vi "CAL_PRESSURE_TRANSDUCER 2016.vi"(7 "Array in":refnum<k24>[](array[refnum]), 8 "error in (no error)":errorcluster, 9 "Descriptions":string[](array[string]), 10 "Sensor Cluster":T1, 11 "pressure_slope_IN":dbl=51.35 format="%.2f") -> (0 "error out":errorcluster, 2 "Sensor Cluster 2":T1, 3 "pressure_slope_OUT":dbl=51.35 format="%.2f", 5 "Array out":refnum<k24>[](array[refnum]))   [LabVIEW 2016]
uses:
  controls/MCC DAQ Readings.ctl
  C:/Program Files (x86)/National Instruments/LabVIEW 2016/vi.lib/ULx/ULx_LV.dll
  Global_SIM_switch.vi
  Kpro Globals.vi
panel:
  out "ok":bool
  out "zero":bool
  out "Pressure":dbl format="%.2f"
  in  "ok":bool
  in  "zero":bool
  # "PRESSURE TRANSDUCER CALIBRATION"
  # "(step 1)"
  # "Fill graduated cylinder to 750 mL water.\nSubmerge Kpro effluent and start flow.\nStop flow at 800 mL of water (1 foot).\nAllow pressure to equilibrate and press zero."
  # "(step 2)"
  # "Hold Kpro effluent facing up and 5' above the floor.\nTurn Kpro flow on briefly to fill the Kpro line.\nTurn Kpro flow off again.\nPress OK when pressure has equilibrated"
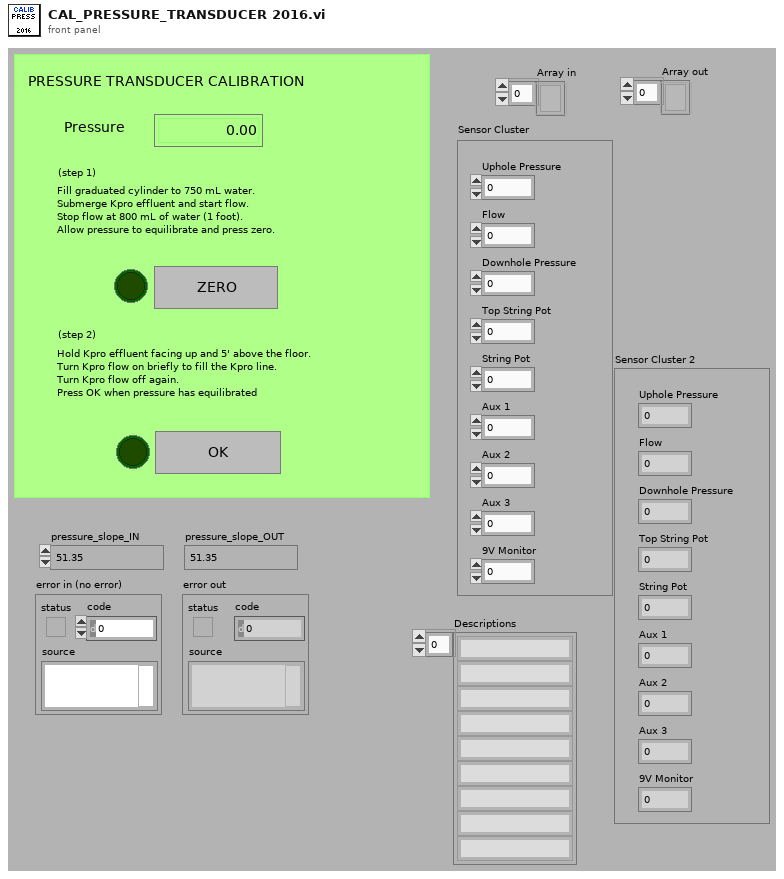
[diagram p1: front panel]
types:
  T1 = typedef "MCC DAQ Readings.ctl" = cluster{"Uphole Pressure":dbl, "Flow":dbl, "Downhole Pressure":dbl, "Top String Pot":dbl, "String Pot":dbl, "Aux 1":dbl, "Aux 2":dbl, "Aux 3":dbl, "9V Monitor":dbl}
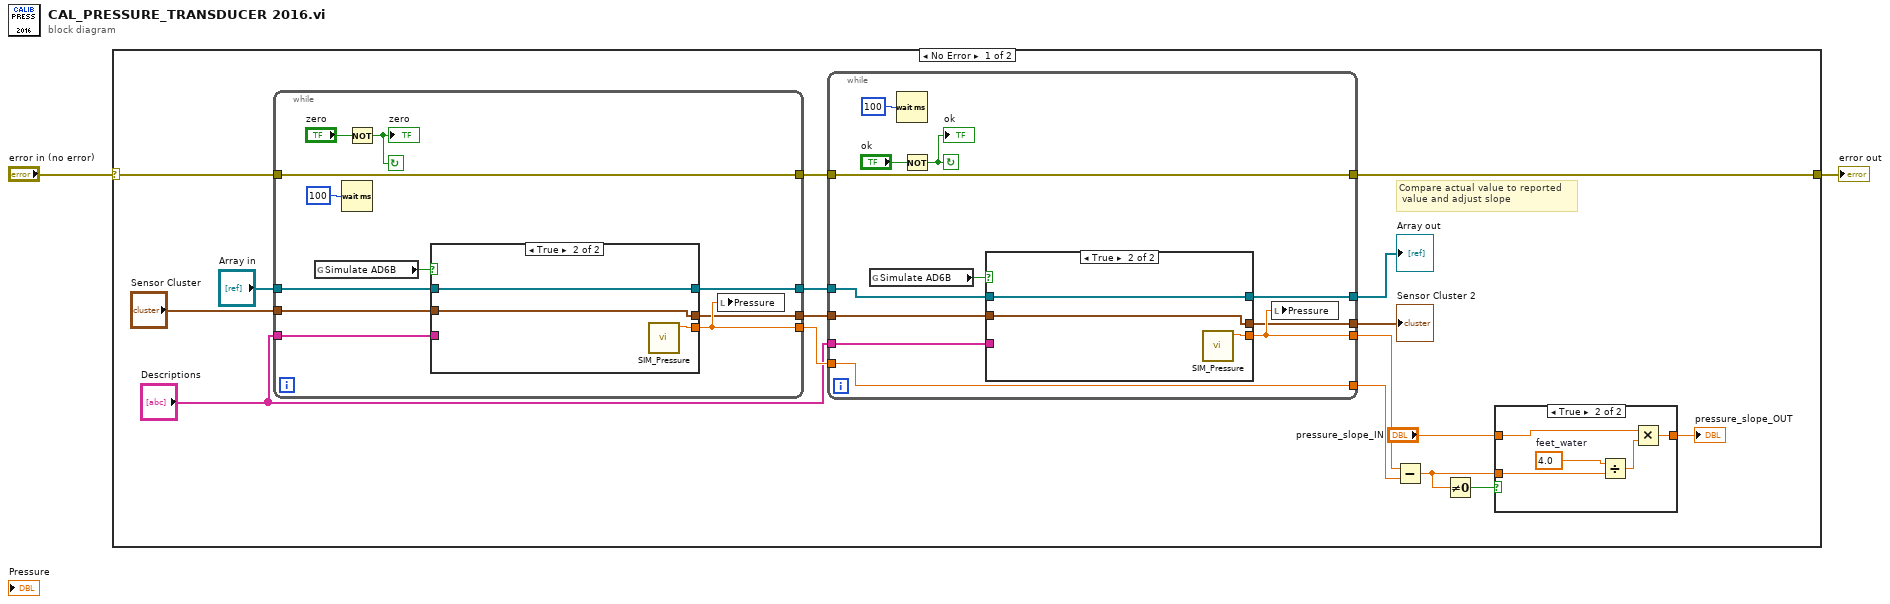
[diagram p0: block diagram]
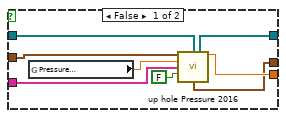
[diagram p3: hidden frame]
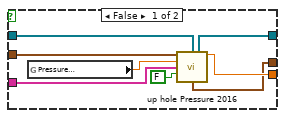
[diagram p4: hidden frame]
diagram:
  n1 = case shown="No Error" "error in (no error)" {
    selector: "error in (no error)" -> [w19 w71]
    tunnel: [w17 w71] -> w2
    frame No Error {
      # "Compare actual value to reported\n value and adjust slope"
      n2 = while {
        tunnel: [w33] -> w13
        tunnel: [w35] -> w18
        tunnel: w19 -> [w35]
        tunnel: "Sensor Cluster" -> [w30]
        tunnel: "Array in" -> [w29]
        tunnel: [w28] -> w11
        tunnel: "Descriptions" -> [w27]
        tunnel: [w26] -> w7
        stop <- w31 continue-if-true
        n3 = global read "Global_SIM_switch.vi" "Simulate AD6B"() -> (w34:bool)
        n4 = Wait (ms)(milliseconds to wait=u32 100) -> ()  [unwired: 1 out]
        n5 = Not(x="zero") -> (.not. x?=w31:bool)
        "zero" <- w31
        n6 = case shown="True" w34 {
          tunnel: [w42 w47] -> w33
          tunnel: w30 -> [w44 w45]
          tunnel: w29 -> [w41 w46]
          tunnel: [w40 w46] -> w28
          tunnel: w27 -> [w39 _]
          tunnel: [w37 w45] -> w26
          frame False {
            n7 = global read "Kpro Globals.vi" "Pressure \nSlope"() -> (w38:dbl)
            n8 = call "up hole Pressure 2016.vi"("Sensor Cluster"=w44, "Array in"=w41, "Pressure \nSlope"=w38, "Descriptions"=w39, "Zero Pressure\n(F = leave as is)"=FALSE ("Zero Pressure\n(F = leave as is)")) -> ("Array out"=w40:refnum<k24>[], "Uphole Pressure"=w42:dbl, "Sensor Cluster 2"=w37:T1)  [unwired: 7 in, 1 out]
          }
          frame True {
            n9 = call "SIM_Pressure.vi"() -> ("Pressure"=w47:dbl)  [unwired: 11 in]
          }
        }
        n10 = local write "Pressure"(w33) -> ()
      }
      n11 = while {
        tunnel: w13 -> [w57]
        tunnel: [w54] -> w14
        tunnel: [w57] -> w16
        tunnel: w18 -> [w58]
        tunnel: [w58] -> w17
        tunnel: w11 -> [w52]
        tunnel: [w51] -> w10
        tunnel: "Descriptions" -> [w50]
        tunnel: w7 -> [w49]
        tunnel: [w48] -> w6
        stop <- w55 continue-if-true
        n12 = global read "Global_SIM_switch.vi" "Simulate AD6B"() -> (w53:bool)
        n13 = Wait (ms)(milliseconds to wait=u32 100) -> ()  [unwired: 1 out]
        n14 = Not(x="ok") -> (.not. x?=w55:bool)
        "ok" <- w55
        n15 = case shown="True" w53 {
          tunnel: [w65 w70] -> w54
          tunnel: w49 -> [w67 w68]
          tunnel: w52 -> [w64 w69]
          tunnel: [w63 w69] -> w51
          tunnel: w50 -> [w62 _]
          tunnel: [w60 w68] -> w48
          frame False {
            n16 = global read "Kpro Globals.vi" "Pressure \nSlope"() -> (w61:dbl)
            n17 = call "up hole Pressure 2016.vi"("Sensor Cluster"=w67, "Array in"=w64, "Pressure \nSlope"=w61, "Descriptions"=w62, "Zero Pressure\n(F = leave as is)"=FALSE ("Zero Pressure\n(F = leave as is)")) -> ("Array out"=w63:refnum<k24>[], "Uphole Pressure"=w65:dbl, "Sensor Cluster 2"=w60:T1)  [unwired: 7 in, 1 out]
          }
          frame True {
            n18 = call "SIM_Pressure.vi"() -> ("Pressure"=w70:dbl)  [unwired: 11 in]
          }
        }
        n19 = local write "Pressure"(w54) -> ()
      }
      "Array out" <- w10
      "Sensor Cluster 2" <- w6
      n20 = Subtract(x=w14, y=w16) -> (x-y=w5:dbl)
      n21 = Not Equal To 0?(x=w5) -> (x != 0?=w3:bool)
      n22 = case shown="True" w3 {
        tunnel: [w20 w24] -> w15
        tunnel: w5 -> [_ w22]
        tunnel: "pressure_slope_IN" -> [w20 w21]
        frame False {
        }
        frame True {
          w25 = 4.0  # feet_water
          n23 = Divide(x=w25, y=w22) -> (x/y=w23:dbl)
          n24 = Multiply(x=w21, y=w23) -> (x*y=w24:dbl)
        }
      }
      "pressure_slope_OUT" <- w15
    }
    frame Error {
    }
  }
  "error out" <- w2
